vi "SA_SPUR_MEAS.vi"() -> ()   [LabVIEW 2018]
panel:
  out "array w/ subset deleted":dbl[](array[numeric])
  in  "Range#":i32=3 min=1 max=20 step=1
  in  "error in":errorcluster {"code" format="%.0x"}
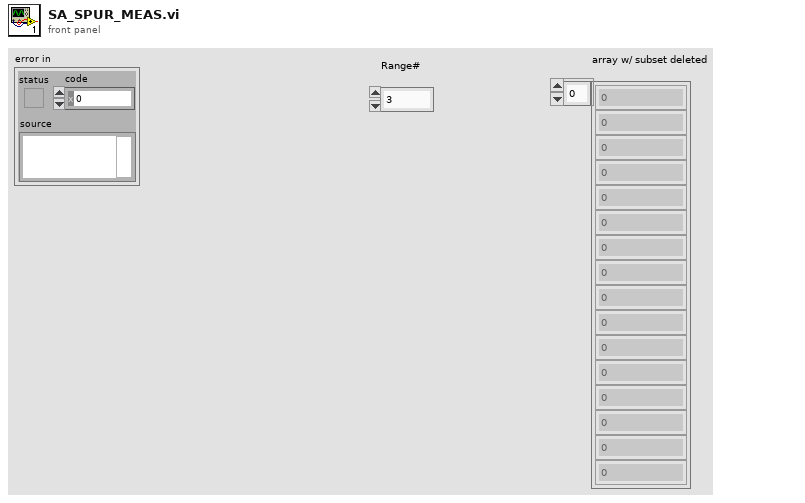
[diagram p1: front panel]
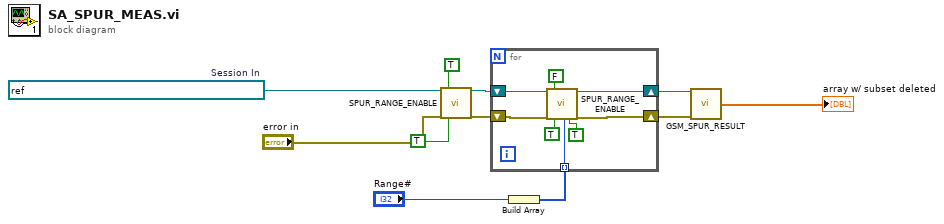
[diagram p0: block diagram]
diagram:
  w7 = refnum<visa-resource-name> "TCPIP0::K-N90X0A-00005.local::inst0::INSTR"  # Session In
  n1 = call "SPUR_RANGE_ENABLE.vi"("Session In"=w7, "error in"="error in", "ALL Ranges OFF"=TRUE, "WRITE"=TRUE) -> ("Session Out"=w11:refnum<visa-resource-name>, "error out"=w10:errorcluster)  [unwired: 14 in]
  n2 = Build Array("Range#") -> (w1:i32[])
  n3 = for {
    tunnel: w1 -> [w15] mode=indexing
    shift-right: [w17] -> w9
    shift-left: w11 -> [w19]
    shift-right: [w16] -> w8
    shift-left: w10 -> [w18]
    n4 = call "SPUR_RANGE_ENABLE.vi"("Session In"=w19, "error in"=w18, "ALL Ranges OFF"=FALSE, "WRITE"=TRUE, "Range#"=w15, "ON/OFF"=TRUE) -> ("Session Out"=w17:refnum<visa-resource-name>, "error out"=w16:errorcluster)  [unwired: 12 in]
  }
  n5 = call "GSM_SPUR_RESULT.vi"("Session In"=w9, "error in"=w8) -> ("array w/ subset deleted"=→"array w/ subset deleted":dbl[])  [unwired: 11 in, 2 out]
